vi "Example v1.vi"() -> ()   [LabVIEW 2020, in "Arduino.lvlib"]
doc: "This example performs writes and reads on a serial port, as directed by the user. You can press the Write and Read buttons, and change the Read Count, while the example is running.\n\nThe parameters set for the serial port must match the parameters of the connected instrument or device. In this example, the Read Count parameter specifies the number of bytes that the serial port reads. If there were more bytes at the port than the specified number, those bytes would not be read. If there were less bytes at the port than the specified number, you would receive a timeout error.\n\nThis example expands upon the flow control options for XON and XOFF, allowing the user to choose those control characters. Also, the user can enable or disable a termination character. Some devices require a termination character in order to identify the end of command strings. Some devices send a termination character to signify the end of data to be read. This example shows how you can end the Read operation once a termination character is detected in the buffer and/or append a termination character at the end of the Write data."
uses:
  Arduino.lvlib
  <vilib>/Instr/_visa.llb/VISA Open Access Mode.ctl
  <vilib>/Instr/_visa.llb/VISA Configure Serial Port (Instr).vi
  <vilib>/National Instruments/Variant Ring Buffer/Ring Buffer.lvclass
panel:
  in  "Scaling":cluster{"K":dbl, "N":dbl}[](array[cluster])=[{"K"=1.0, "N"=0.0}, {"K"=1.0, "N"=0.0}, {"K"=100.0, "N"=0.0}, {"K"=100.0, "N"=0.0}, {"K"=1.0, "N"=0.0}, {"K"=1.0, "N"=0.0}]
  in  "Serial Settings":T1={"baud rate"=115200, "data bits"=8, "parity"=enum."None", "stop bits"=10, "flow control"=0} {"flow control" items=["None"=0, "XON/XOFF"=1, "RTS/CTS"=2, "DTR/DSR"=4]; "stop bits" items=["1.0"=10, "1.5"=15, "2.0"=20]; "data bits" min=5 max=8 step=1; "baud rate" items=["75"=75, "110"=110, "134"=134, "150"=150, "300"=300, "600"=600, "1200"=1200, "1800"=1800, "2400"=2400, "4800"=4800, "7200"=7200, "9600"=9600, "14400"=14400, "19200"=19200, "28800"=28800, "38400"=38400, "56000"=56000, "57600"=57600, "115200"=115200, "128000"=128000, "230400"=230400]}
  out "length":i32=246
  out "Chart":dbl[][](graph)
  out "Number of Bytes at Serial Port":u32=246
  in  "Stop":bool
  out "Response":string="519 \t519 \t518 \t518 \t518 \t518 \t518 \t519 \t518 \t518\t1023 \t1023 \t1023 \t1023 \t1023 \t1023 \t1023 \t1023 \t1023 \t1023\t45 \t45 \t45 \t45 \t46 \t45 \t46 \t45 \t46 \t46\t63 \t63 \t63 \t62 \t63 \t63 \t62 \t63 \t62 \t63\t0 \t1 \t0 \t1 \t0 \t1 \t0 \t0 \t1 \t1\t0 \t0 \t1 \t0 \t1 \t1 \t1 \t0 \t1 \t0\t\r\n"
  in  "VISA resource name":refnum<visa-resource-name>="COM3"
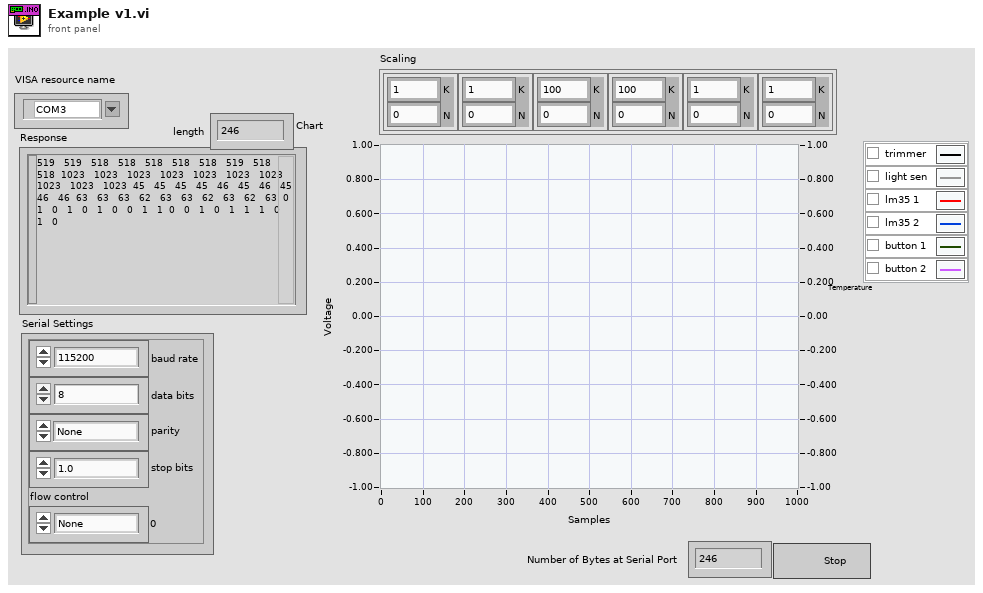
[diagram p1: front panel]
types:
  T1 = cluster{"baud rate":u32, "data bits":u16, "parity":enum16{"None", "Odd", "Even", "Mark", "Space"}, "stop bits":u16, "flow control":u16}
  T2 = typedef "VISA Open Access Mode.ctl" = u32
  T3 = cluster{"XON":enum16{"NUL", "SOH", "STX", "ETX", "EOT", "ENQ", "ACK", "BEL", "BS", "HT", "LF", "VT", "FF", "CR", "SO", "SI", "DLE", "DC1", "DC2", "DC3", "DC4", "NAK", "SYN", "ETB", "CAN", "EM", "SUB", "ESC", "FS", "GS", "RS", "US", "SP", "!", "\"", "#", "$", "%", "&", "'", "(", ")", "*", "+", ",", "- (-)", ".", "/", "0", "1", "2", "3", "4", "5", "6", "7", "8", "9", ":", ";", "<", "=", ">", "?", "@", "A", "B", "C", "D", "E", "F", "G", "H", "I", "J", "K", "L", "M", "N", "O", "P", "Q", "R", "S", "T", "U", "V", "W", "X", "Y", "Z", "[", "\\", "]", "^", "_", "`", "a", "b", "c", "d", "e", "f", "g", "h", "i", "j", "k", "l", "m", "n", "o", "p", "q", "r", "s", "t", "u", "v", "w", "x", "y", "z", "{", "|", "}", "~"}, "XOFF":enum16{"NUL", "SOH", "STX", "ETX", "EOT", "ENQ", "ACK", "BEL", "BS", "HT", "LF", "VT", "FF", "CR", "SO", "SI", "DLE", "DC1", "DC2", "DC3", "DC4", "NAK", "SYN", "ETB", "CAN", "EM", "SUB", "ESC", "FS", "GS", "RS", "US", "SP", "!", "\"", "#", "$", "%", "&", "'", "(", ")", "*", "+", ",", "- (-)", ".", "/", "0", "1", "2", "3", "4", "5", "6", "7", "8", "9", ":", ";", "<", "=", ">", "?", "@", "A", "B", "C", "D", "E", "F", "G", "H", "I", "J", "K", "L", "M", "N", "O", "P", "Q", "R", "S", "T", "U", "V", "W", "X", "Y", "Z", "[", "\\", "]", "^", "_", "`", "a", "b", "c", "d", "e", "f", "g", "h", "i", "j", "k", "l", "m", "n", "o", "p", "q", "r", "s", "t", "u", "v", "w", "x", "y", "z", "{", "|", "}", "~"}}
  T4 = enum16{"NUL", "SOH", "STX", "ETX", "EOT", "ENQ", "ACK", "BEL", "BS", "HT", "LF", "VT", "FF", "CR", "SO", "SI", "DLE", "DC1", "DC2", "DC3", "DC4", "NAK", "SYN", "ETB", "CAN", "EM", "SUB", "ESC", "FS", "GS", "RS", "US", "SP", "!", "\"", "#", "$", "%", "&", "'", "(", ")", "*", "+", ",", "- (-)", ".", "/", "0", "1", "2", "3", "4", "5", "6", "7", "8", "9", ":", ";", "<", "=", ">", "?", "@", "A", "B", "C", "D", "E", "F", "G", "H", "I", "J", "K", "L", "M", "N", "O", "P", "Q", "R", "S", "T", "U", "V", "W", "X", "Y", "Z", "[", "\\", "]", "^", "_", "`", "a", "b", "c", "d", "e", "f", "g", "h", "i", "j", "k", "l", "m", "n", "o", "p", "q", "r", "s", "t", "u", "v", "w", "x", "y", "z", "{", "|", "}", "~"}
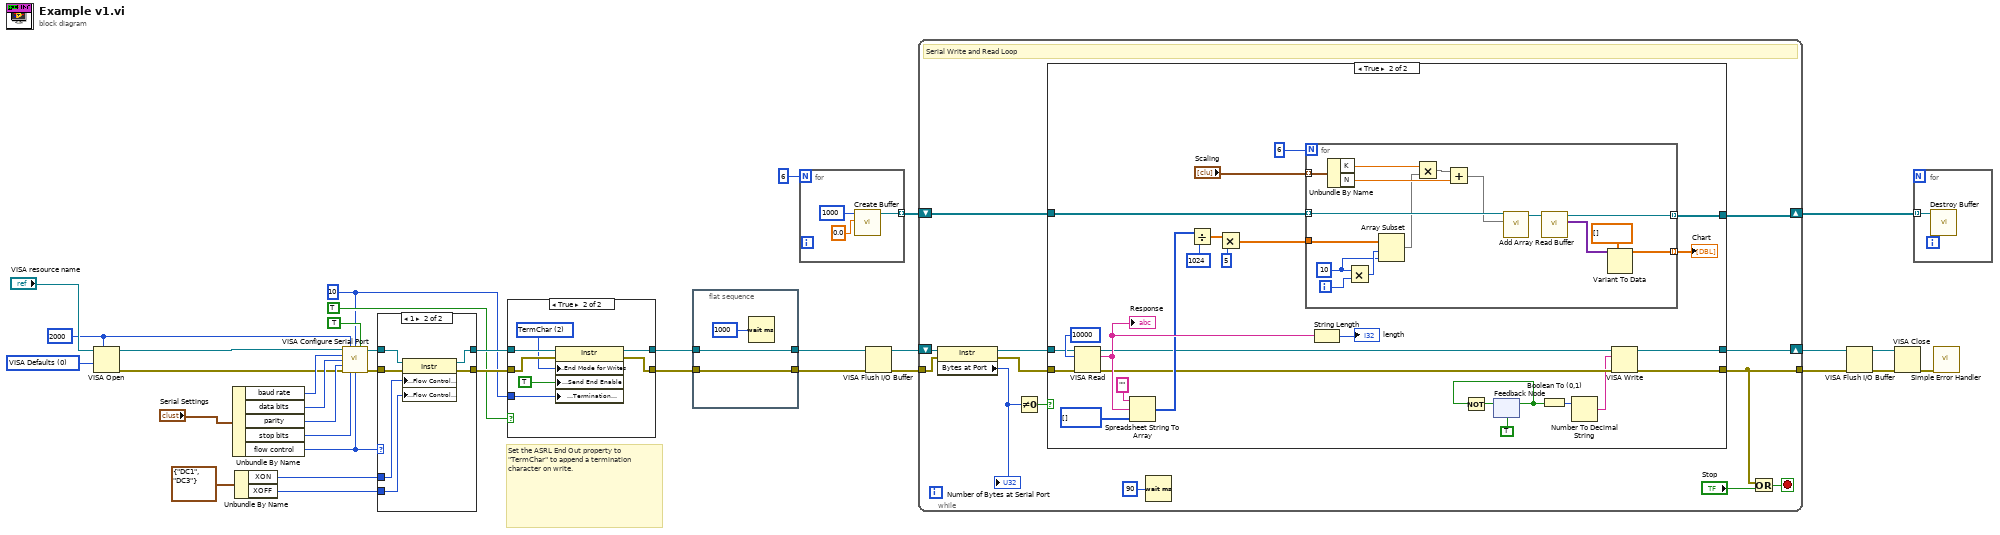
[diagram p0: block diagram]
diagram:
  w1 = u32 2000 ("VISA Open timeout (0)")
  w2 = T2 0 items=["VISA Defaults"=0, "Exclusive Lock"=1, "Load Configured Settings"=4] ("Access Mode")
  w19 = u8 10 ("Termination Character")
  # "Set the ASRL End Out property to \"TermChar\" to append a termination character on write."
  n1 = VISA Open(timeout (0)=w1, access mode=w2, VISA resource name="VISA resource name") -> (VISA resource name=w4:refnum<visa-resource-name>, error out=w3:errorcluster)  [unwired: 2 in]
  n2 = Unbundle By Name("Serial Settings") -> ("baud rate"=w29:u32, "data bits"=w30:u16, "parity"=w31:enum16{"None", "Odd", "Even", "Mark", "Space"}, "stop bits"=w32:u16, "flow control"=w25:u16)
  n3 = Unbundle By Name(T3 {"XON"=enum."DC1", "XOFF"=enum."DC3"} ("XON/XOFF Characters")) -> ("XON"=w24:T4, "XOFF"=w23:T4)
  n4 = call-poly "VISA Configure Serial Port"("VISA resource name"=w4, "timeout (10sec)"=w1, "termination char\n(0xA = '\\n' = LF)"=w19, "Enable Termination\nChar (T)"=TRUE ("End Read on Termination Character?"), "baud rate (9600)"=w29, "data bits (8)"=w30, "parity (0:none)"=w31, "error in (no error)"=w3, "stop bits (10: 1 bit)"=w32, "flow control (0:none)"=w25) -> ("VISA resource name out"=w33:refnum<visa-resource-name>, "error out"=w34:errorcluster)  [unwired: 4 out]
  n5 = case shown="1" w25 {
    tunnel: [w36 w43] -> w22
    tunnel: [w37 w42] -> w21
    tunnel: w34 -> [w36 w41]
    tunnel: w33 -> [w37 w40]
    tunnel: w24 -> [_ w39]
    tunnel: w23 -> [_ w38]
    frame Default {
    }
    frame 1 {
      n6 = property class="Instr"(reference=w40, error in=w41, "Serial Settings:Flow Control XON Character"=w39, "Serial Settings:Flow Control XOFF Character"=w38) -> (reference out=w42:refnum<visa-resource-name>, error out=w43:errorcluster)
    }
  }
  n7 = case shown="True" TRUE ("End Write on Termination Character?") {
    tunnel: w21 -> [w44 w52]
    tunnel: w22 -> [w45 w51]
    tunnel: [w44 w50] -> w18
    tunnel: [w45 w49] -> w17
    tunnel: w19 -> [_ w47]
    frame False {
    }
    frame True {
      w48 = u16 2 items=["None", "LastBit", "TermChar", "Break"] ("Serial Settings:Serial End Mode for Writes")
      n8 = property class="Instr"(reference=w52, error in=w51, "Serial Settings:End Mode for Writes"=w48, "Message Based Settings:Send End Enable"=TRUE, "Message Based Settings:Termination Character"=w47) -> (reference out=w50:refnum<visa-resource-name>, error out=w49:errorcluster)
    }
  }
  n9 = flat-sequence {
    tunnel: [w55] -> w7
    tunnel: w18 -> [w55]
    tunnel: [w54] -> w6
    tunnel: w17 -> [w54]
    frame #0 {
      n10 = Wait (ms)(milliseconds to wait=u32 1000) -> ()  [unwired: 1 out]
    }
  }
  n11 = for {
    N: 6 -> [_]
    tunnel: [w56] -> w14 mode=indexing
    n12 = call <vilib>:"Create Buffer.vi"("Data Type"=0.0, "Buffer Size"=1000) -> ("Ring Buffer Reference"=w56:refnum<data-value>)  [unwired: 8 in, 1 out]
  }
  n13 = VISA Flush I/O Buffer(VISA resource name=w7, error in (no error)=w6) -> (VISA resource name out=w16:refnum<visa-resource-name>, error out=w15:errorcluster)  [unwired: 1 in]
  n14 = while {
    shift-right: [w71] -> w11
    shift-left: w16 -> [w66]
    tunnel: w15 -> [w61]
    tunnel: [w68] -> w9
    shift-right: [w59] -> w13
    shift-left: w14 -> [w60]
    stop <- w69 stop-if-true
    # "Serial Write and Read Loop"
    n15 = property class="Instr"(reference=w66, error in=w61) -> (reference out=w65:refnum<visa-resource-name>, error out=w62:errorcluster, "Bytes at Port"=w64:u32)
    "Number of Bytes at Serial Port" <- w64
    n16 = Not Equal To 0?(x=w64) -> (x != 0?=w63:bool)
    n17 = case shown="True" w63 {
      tunnel: [w74 w82] -> w71
      tunnel: w62 -> [w73 w100]
      tunnel: [w73 w80] -> w68
      tunnel: w65 -> [w74 w98]
      tunnel: w60 -> [w72 w92]
      tunnel: [w72 w90] -> w59
      frame False {
      }
      frame True {
        n18 = VISA Read(VISA resource name=w98, byte count=u32 10000 ("Read Count"), error in (no error)=w100) -> (VISA resource name out=w83:refnum<visa-resource-name>, read buffer=w94:string, error out=w81:errorcluster)  [unwired: 1 out]
        "Response" <- w94
        n19 = Spreadsheet String To Array(format string="", spreadsheet string=w94, array type (2D Dbl)=i32[] []) -> (array=w85:i32[])  [unwired: 1 in]
        n20 = Divide(x=w85, y=1024) -> (x/y=w88:dbl[])
        n21 = Multiply(x=w88, y=5) -> (x*y=w86:dbl[])
        n22 = for {
          N: 6 -> [_]
          tunnel: w86 -> [w116]
          tunnel: w92 -> [w112] mode=indexing
          tunnel: [w110] -> w90 mode=indexing
          tunnel: [w107] -> w91 mode=indexing
          tunnel: "Scaling" -> [w106] mode=indexing
          i -> [w115]
          w113 = 10 ("x")
          n23 = Unbundle By Name(w106) -> ("K"=w105:dbl, "N"=w103:dbl)
          n24 = Multiply(x=w113, y=w115) -> (x*y=w114:i32)
          n25 = Array Subset(array=w116, index=w114, length=w113) -> (w102:dbl[])
          n26 = Multiply(x=w105, y=w102) -> (x*y=w104:dbl[])
          n27 = Add(x=w104, y=w103) -> (x+y=w101:dbl[])
          n28 = call <vilib>:"Add Array.vi"("Variants Array"=w101, "Ring Buffer Reference"=w112) -> ("Ring Buffer Reference"=w111:refnum<data-value>)  [unwired: 8 in, 1 out]
          n29 = call <vilib>:"Read Buffer.vi"("Ring Buffer Reference"=w111) -> ("Array of Variants"=w109:variant[], "Ring Buffer Reference"=w110:refnum<data-value>)  [unwired: 8 in, 1 out]
          n30 = Variant To Data(type=dbl[] [] ("subarray"), Variant=w109) -> (data=w107:dbl[])  [unwired: 1 in, 1 out]
        }
        "Chart" <- w91
        n31 = String Length(string=w94) -> (length=→"length":i32)
        n32 = feedback #1(TRUE) -> (w75:bool)
        n33 = Not(x=w75) -> (.not. x?=w76:bool)
        n34 = feedback-in #1(w76) -> ()
        n35 = Boolean To (0,1)(Boolean=w75) -> (0, 1=w78:i16)
        n36 = Number To Decimal String(number=w78) -> (decimal integer string=w79:string)  [unwired: 1 in]
        n37 = VISA Write(VISA resource name=w83, write buffer=w79, error in (no error)=w81) -> (VISA resource name out=w82:refnum<visa-resource-name>, error out=w80:errorcluster)  [unwired: 1 out]
      }
    }
    n38 = Wait (ms)(milliseconds to wait=u32 90) -> ()  [unwired: 1 out]
    n39 = Or(x=w68, y="Stop") -> (x .or. y?=w69:bool)
  }
  n40 = VISA Flush I/O Buffer(VISA resource name=w11, error in (no error)=w9) -> (VISA resource name out=w10:refnum<visa-resource-name>, error out=w8:errorcluster)  [unwired: 1 in]
  n41 = VISA Close(VISA resource name=w10, error in (no error)=w8) -> (error out=w26:errorcluster)
  n42 = for {
    tunnel: w13 -> [w117] mode=indexing
    n43 = call <vilib>:"Destroy Buffer.vi"("Ring Buffer Reference"=w117) -> ()  [unwired: 9 in, 2 out]
  }
  n44 = call <vilib>:"Simple Error Handler.vi"("error in (no error)"=w26) -> ()  [unwired: 1 in, 8 out]
